vi "String.Append Item to String List.vi"(5 "Delimiter":string=", ", 7 "Prefix":string, 10 "New Data":string, 11 "Existing Str":string) -> (3 "New Str":string)   [LabVIEW 2024]
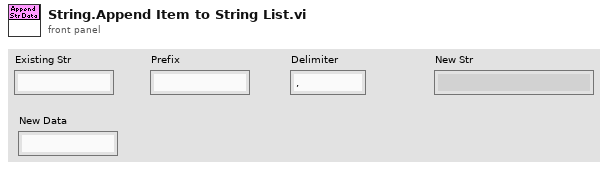
[diagram p1: front panel]
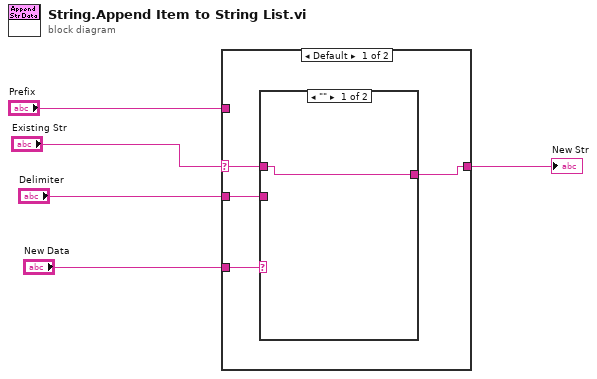
[diagram p0: block diagram]
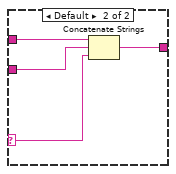
[diagram p2: hidden frame]
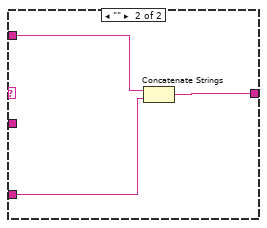
[diagram p3: hidden frame]
diagram:
  n1 = case shown="Default" "Existing Str" {
    selector: "Existing Str" -> [w9 _]
    tunnel: [w7 w16] -> w3
    tunnel: "New Data" -> [w8 w17]
    tunnel: "Prefix" -> [_ w15]
    tunnel: "Delimiter" -> [w6 _]
    frame Default {
      n2 = case shown="\"\"" w8 {
        selector: w8 -> [_ w13]
        tunnel: w9 -> [w10 w14]
        tunnel: [w10 w12] -> w7
        tunnel: w6 -> [_ w11]
        frame "" {
        }
        frame Default {
          n3 = Concatenate Strings(w14, w11, w13) -> (w12:string)
        }
      }
    }
    frame "" {
      n4 = Concatenate Strings(w15, w17) -> (w16:string)
    }
  }
  "New Str" <- w3
